vi "Get Next Test.vi"(8 "error in (no error)":errorcluster, 9 "Active Unique ID":string, 11 "Test Executive in":refnum<class "Test Executive.lvclass">) -> (0 "error out":errorcluster, 1 "Active Unique ID out":string, 2 "Test":refnum<class "Executioner.lvclass">, 3 "Test Executive out":refnum<class "Test Executive.lvclass">, 4 "Found":bool, 5 "Test Executive Ref out":refnum<data-value>, 6 "Complete":bool)   [LabVIEW 2019, in "Test Executive.lvlib" / "Test Executive.lvclass"]
uses:
  <vilib>/gpm_packages/@cs/test-executive/Source/Test Executive/TestExecutive/Test Executive.lvclass
  <vilib>/gpm_packages/@cs/test-executive/Source/Test Executive/Executioner/Executioner.lvclass
  <vilib>/gpm_packages/@cs/test-executive/Source/Test Executive/ITestExecutive/ITest Executive.lvclass
  <vilib>/gpm_packages/@cs/test-executive/Source/Test Executive/TestExecutive/Test Executive.lvclass/Test Executive.ctl
  <vilib>/gpm_packages/@cs/linked-list/Source/Linked List/Linked List Ref/Linked List Ref.lvclass
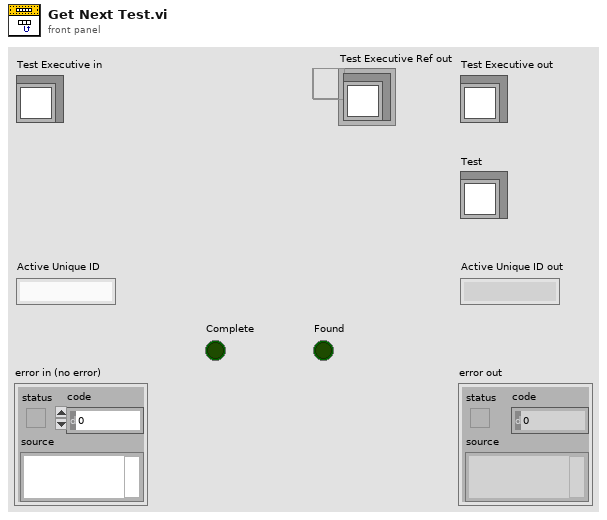
[diagram p1: front panel]
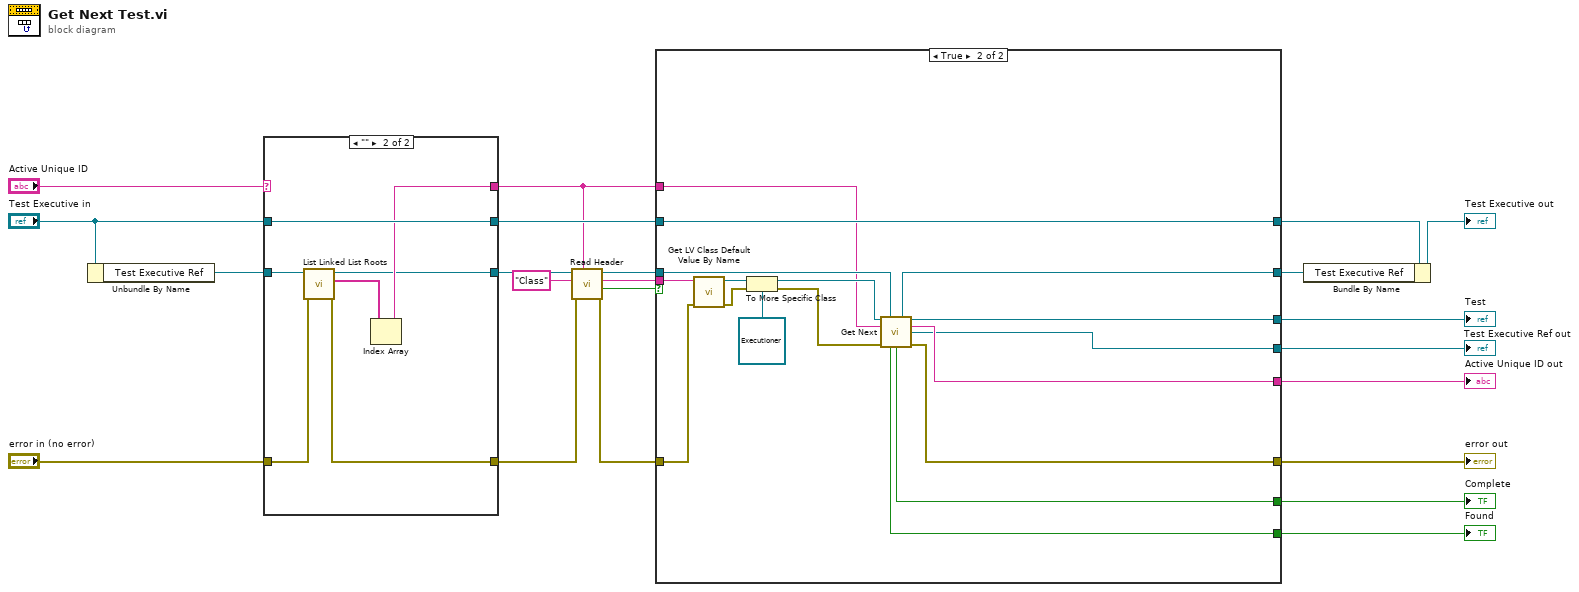
[diagram p0: block diagram]
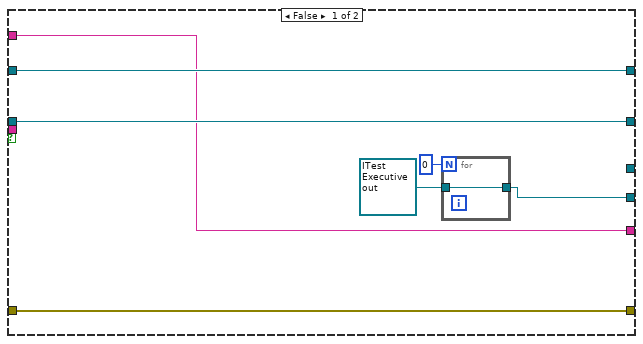
[diagram p2: hidden frame]
diagram:
  n1 = Unbundle By Name("Test Executive in") -> ("Test Executive Ref"=w21:refnum<data-value>)
  n2 = case shown="\"\"" "Active Unique ID" {
    selector: "Active Unique ID" -> [w25 _]
    tunnel: "Test Executive in" -> [w26 w33]
    tunnel: w21 -> [w24 w32]
    tunnel: [w26 w33] -> w11
    tunnel: "error in (no error)" -> [w23 w31]
    tunnel: [w25 w29] -> w6
    tunnel: [w24 w28] -> w18
    tunnel: [w23 w27] -> w14
    frame Default {
    }
    frame "" {
      n3 = call <vilib>:"List Linked List Roots.vi"("error in (no error)"=w31, "Linked List Ref"=w32) -> ("error out"=w27:errorcluster, "Root IDs"=w30:string[], "Linked List Ref out"=w28:refnum<data-value>)  [unwired: 6 in, 1 out]
      n4 = Index Array(array=w30) -> (element=w29:string)  [unwired: 1 in]
    }
  }
  n5 = call <vilib>:"Read Header.vi"("Linked List ID"=w6, "error in (no error)"=w14, "Header Name"="Class", "Linked List Ref"=w18) -> ("error out"=w15:errorcluster, "found"=w16:bool, "Header Value"=w12:string, "Linked List Ref out"=w13:refnum<data-value>)  [unwired: 4 in]
  n6 = case shown="True" w16 {
    tunnel: w15 -> [w38 w55]
    tunnel: w13 -> [w39 w53]
    tunnel: w12 -> [_ w58]
    tunnel: w11 -> [w40 w48]
    tunnel: [w40 w48] -> w8
    tunnel: [w39 w45] -> w10
    tunnel: [w38 w44] -> w7
    tunnel: w6 -> [w37 w47]
    tunnel: [_ w46] -> w5
    tunnel: [w37 w51] -> w4
    tunnel: [_ w50] -> w3
    tunnel: [_ w42] -> w2
    tunnel: [w34 w43] -> w1
    frame False {
      n7 = for {
        N: 0 -> [_]
        tunnel: refnum<data-value> refnum ("Test Executive Ref out") -> [w41]
        tunnel: [w41] -> w34
      }
    }
    frame True {
      n8 = call <vilib>:"Get LV Class Default Value By Name.vi"("error in (no error)"=w55, "class name"=w58) -> ("error out"=w54:errorcluster, "object"=w57:refnum<class>)  [unwired: 8 in]
      n9 = To More Specific Class(target class=refnum<class "Executioner.lvclass"> refnum ("Test Executive.lvlib:Executioner.lvclass"), reference=w57, error in=w54) -> (specific class reference=w49:refnum<class "Executioner.lvclass">, error out=w52:errorcluster)
      n10 = call-dynamic "Get Next.vi"("Executioner in"=w49, "Linked List Ref"=w53, "Active Unique ID"=w47, "error in (no error)"=w52) -> ("Linked List Ref out"=w45:refnum<data-value>, "Executioner out"=w46:refnum<class "Executioner.lvclass">, "Active Unique ID out"=w51:string, "Test Executive Ref out"=w43:refnum<data-value>, "Found"=w50:bool, "Complete"=w42:bool, "error out"=w44:errorcluster)  [unwired: 3 in, 2 out]
    }
  }
  "error out" <- w7
  "Active Unique ID out" <- w4
  "Test" <- w5
  "Found" <- w3
  "Complete" <- w2
  "Test Executive Ref out" <- w1
  n11 = Bundle By Name(cluster=w8, "Test Executive Ref"=w10) -> (→"Test Executive out":refnum<class "Test Executive.lvclass">)
